vi "ProdaNG.Tree.WabcoPart.Clear.vi"(7 "Tree":refnum<vi>, 8 "error in (no error)":errorcluster, 10 "Tag":string) -> (0 "error out":errorcluster)   [LabVIEW 2016]
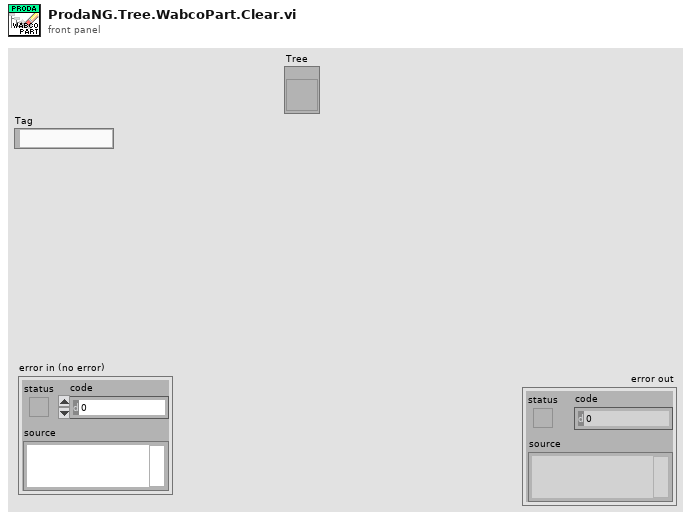
[diagram p1: front panel]
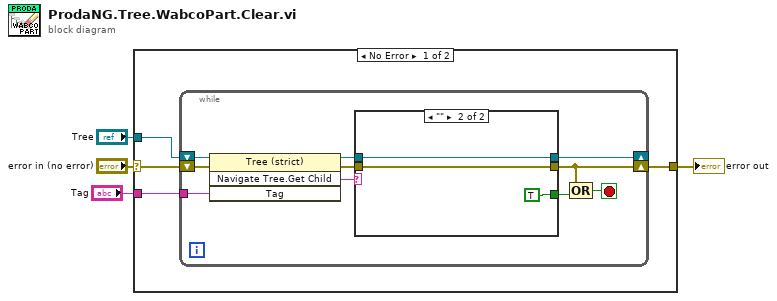
[diagram p0: block diagram]
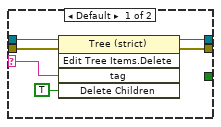
[diagram p2: hidden frame]
diagram:
  n1 = case shown="No Error" "error in (no error)" {
    selector: "error in (no error)" -> [w7 w28]
    tunnel: [w5 w28] -> w3
    tunnel: "Tree" -> [w6 _]
    tunnel: "Tag" -> [w8 _]
    frame No Error {
      n2 = while {
        shift-right: [w12] -> _
        shift-left: w6 -> [w18]
        shift-right: [w11] -> w5
        shift-left: w7 -> [w16]
        tunnel: w8 -> [w17]
        stop <- w10 stop-if-true
        n3 = invoke class="Tree (strict)" method="Navigate Tree.Get Child"(reference=w18, error in=w16, "Tag"=w17) -> (reference out=w15:refnum<vi>, error out=w14:errorcluster, "Navigate Tree:Get Child"=w13:string)  [unwired: 1 in, 1 out]
        n4 = case shown="\"\"" w13 {
          selector: w13 -> [w22 _]
          tunnel: w15 -> [w24 w27]
          tunnel: w14 -> [w23 w26]
          tunnel: [w21 w27] -> w12
          tunnel: [w20 w26] -> w11
          tunnel: [_ TRUE] -> w9
          frame Default {
            n5 = invoke class="Tree (strict)" method="Edit Tree Items.Delete"(reference=w24, error in=w23, "tag"=w22, "Delete Children"=TRUE ("Delete Children?")) -> (reference out=w21:refnum<vi>, error out=w20:errorcluster)  [unwired: 1 in, 3 out]
          }
          frame "" {
          }
        }
        n6 = Compound Arithmetic op=OR(w11, w9) -> (w10:bool)
      }
    }
    frame Error {
    }
  }
  "error out" <- w3
